vi "Vision Data.vi"() -> ()   [LabVIEW 2014]
panel:
  in  "Y":dbl
  in  "X":dbl
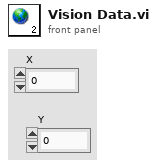
[diagram p1: front panel]
diagram:
